vi "SetSelectionMode.vi"(0 "reference in":refnum<class "DataGridView.lvclass">, 5 "SelectionMode":i32(ring) items=["CellSelect", "FullRowSelect", "FullColumnSelect", "RowHeaderSelect", "ColumnHeaderSelect"], 7 "MultiSelect":bool, 11 "error in (no error)":errorcluster) -> (4 "reference out":refnum<class "DataGridView.lvclass">, 15 "error out":errorcluster)   [LabVIEW 2018, in "DataGridView.lvclass"]
doc: "Set the selection mode of the DataGridView"
uses:
  DataGridView.lvclass
  System.Windows.Forms
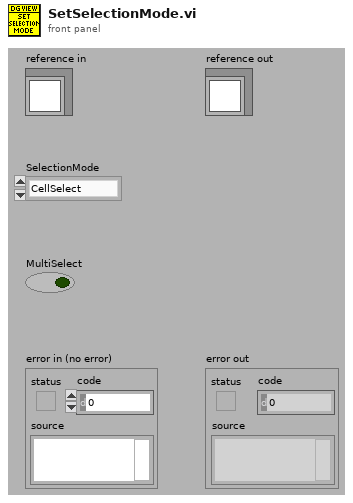
[diagram p1: front panel]
types:
  T1 = typedef "DataGridView.lvclass/ObjectAttributes.ctl" = cluster{"DataGridView":refnum<k24>, "SelectionChangedEvent":refnum<user-event>, "SelectionChanged callback ref":refnum<k27>, "LastSelectedRowIndex":i32}
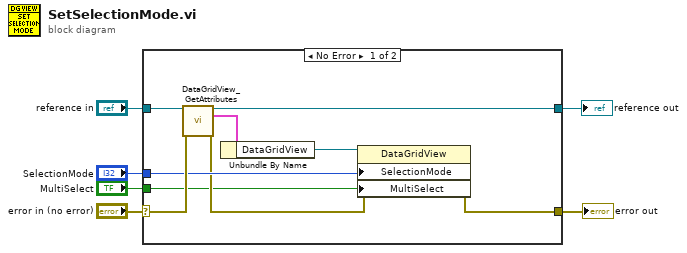
[diagram p0: block diagram]
diagram:
  n1 = case shown="No Error" "error in (no error)" {
    selector: "error in (no error)" -> [w15 w17]
    tunnel: [w8 w17] -> w5
    tunnel: [w12 w16] -> w3
    tunnel: "reference in" -> [w13 w16]
    tunnel: "SelectionMode" -> [w10 _]
    tunnel: "MultiSelect" -> [w7 _]
    frame No Error {
      n2 = call "DataGridView_GetAttributes.vi"("reference in"=w13, "error in (no error)"=w15) -> ("reference out"=w12:refnum<class "DataGridView.lvclass">, "Data"=w14:T1, "error out"=w9:errorcluster)  [unwired: 10 in, 1 out]
      n3 = Unbundle By Name(w14) -> ("DataGridView"=w11:refnum<k24>)
      n4 = property class="DataGridView"(reference=w11, error in=w9, "SelectionMode"=w10, "MultiSelect"=w7) -> (error out=w8:errorcluster)  [unwired: 1 out]
    }
    frame Error {
    }
  }
  "error out" <- w5
  "reference out" <- w3
